vi "SL TAGS Write Server Tag.vi"(8 "error in (no error)":errorcluster, 10 "Value":variant, 11 "Tag Ref In":T1) -> (0 "error out":errorcluster, 3 "Tag Ref Out":T1)   [LabVIEW 2017, in "EEISysLink.lvclass"]
doc: "Will input a class tag and write its value to the SystemLink server. \n\nNote: this does not update the local class tag value. You must read from the server to get the value. \n\nJames Tillett P.E.\nEndeavor Engineering Inc.\nwww.endeavoreng.com"
uses:
  EEISysLink.lvclass
  Controls/SL Tag.ctl
  <vilib>/Skyline/Tag/Wrapper/Wrapper_class/NI Skyline Tag.lvclass
  Controls/SL Tag Properties.ctl
  Controls/SL Tag Data Type.ctl
  Controls/SL Tag Interpolation Method.ctl
  Controls/SL Tag Unit of Measure.ctl
  Controls/SL Tag Type.ctl
  <vilib>/Skyline/Tag/Shared/typedefs/Tag Cluster.ctl
  <vilib>/Skyline/Tag/Shared/typedefs/DataType.ctl
  <vilib>/Skyline/Tag/Wrapper/Wrapper_class/Write Tag (DBL).vi
  <vilib>/Skyline/Tag/Wrapper/Wrapper_class/Write Tag (I32).vi
  <vilib>/Skyline/Tag/Wrapper/Wrapper_class/Write Tag (String).vi
  <vilib>/Skyline/Tag/Shared/NI Skyline Tag.lvlib
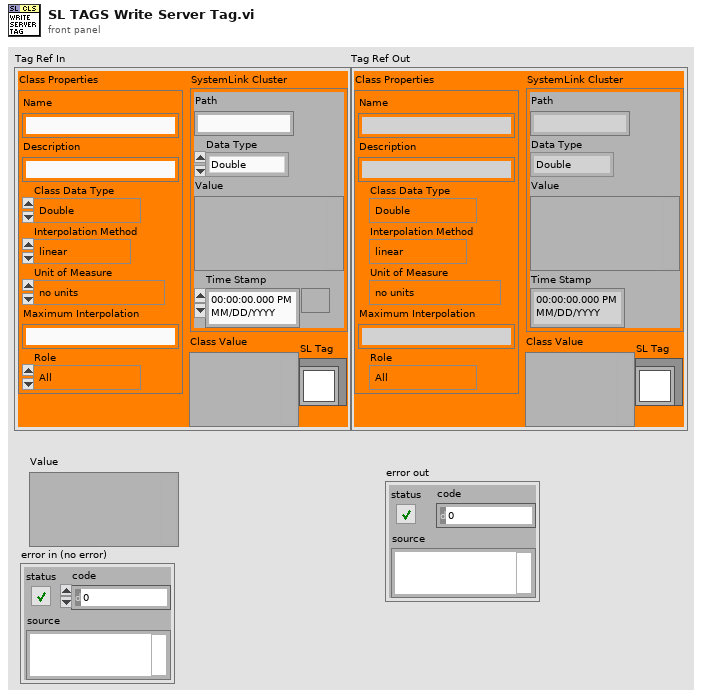
[diagram p1: front panel]
types:
  T1 = typedef "EEISysLink.lvclass/SL Tag.ctl" = cluster{"Class Properties":T2, "SL Tag":refnum<class "NI Skyline Tag.lvclass">, "SystemLink Cluster":T7, "Class Value":variant}
  T2 = typedef "EEISysLink.lvclass/SL Tag Properties.ctl" = cluster{"Class Data Type":T3, "Name":string, "Description":string, "Interpolation Method":T4, "Unit of Measure":T5, "Maximum Interpolation":string, "Role":T6}
  T3 = typedef "EEISysLink.lvclass/SL Tag Data Type.ctl" = enum16{"Double", "Integer", "String", "Boolean", "Waveform"}
  T4 = typedef "EEISysLink.lvclass/SL Tag Interpolation Method.ctl" = enum16{"linear", "pilinear", "step"}
  T5 = typedef "EEISysLink.lvclass/SL Tag Unit of Measure.ctl" = enum16{"no units", "Second", "Hour", "Minute", "Day", "Year", "Month", "Week", "Foot", "Yard", "Meter", "Centimeter", "Inch", "Mile", "Nautical Mile", "Miles per Hour", "Meters per second", "Square meter", "Cubic meter", "Cubic centimeter", "Cubic inch", "Liter", "Gallon", "Gallons dry US", "Gallon UK", "Percent", "Revolutions per minute", "Revolution", "Degree angle", "Astronomical Unit", "Atom", "Atomic mass", "Bar", "Byte", "C (speed of light)", "Curie", "Decibel", "Electron Volt", "Ounce", "Knot", "G", "Grade", "Are", "Hectare", "Faraday", "Franklin", "Gilbert", "Erg", "Lambert", "Maxwell", "Gauss", "Electron mass", "Kilogram force", "Pound force", "Rad", "Centiradian", "Sphere", "Mach", "Fluid Ounces", "Fluid Ounces UK", "Fahrenheit", "Celsius", "Kelvin", "Rankine", "Gram", "Kilogram", "Pound", "Short/US Ton", "Long/UK ton", "Metric ton", "Mole", "Pounds per square inch", "Inches water column", "Torr", "Millitorr", "Millimeter mercury", "Inches mercury", "Bar (2)", "Atmosphere", "Pascal", "Watt", "kiloWatt", "Horsepower", "Kilowatt Hour", "British thermal units", "Millions of BTU", "Ampere", "Candela", "Radian", "Steradian", "Bit", "Hertz", "Newton", "Joule", "Coulomb", "Volt", "Farad", "Ohm", "Siemens", "Weber", "Tesla", "Henry", "Lumen", "Lux", "Becqueral", "Gray", "Sievert", "Katal", "Angstrom", "Light Year", "Parsec", "Point", "Pixel", "Dyne", "Kilogram force (2)", "Pound force (2)", "Rem", "Rutherford", "Roentgen"}
  T6 = typedef "EEISysLink.lvclass/SL Tag Type.ctl" = enum16{"All", "Supervisor", "Worker"}
  T7 = typedef "NI Skyline Tag.lvlib/Tag Cluster.ctl" = cluster{"Path":string, "Data Type":T8, "Value":variant, "Time Stamp":timestamp}
  T8 = typedef "NI Skyline Tag.lvlib/DataType.ctl" = enum32{"Double", "Integer", "String"}
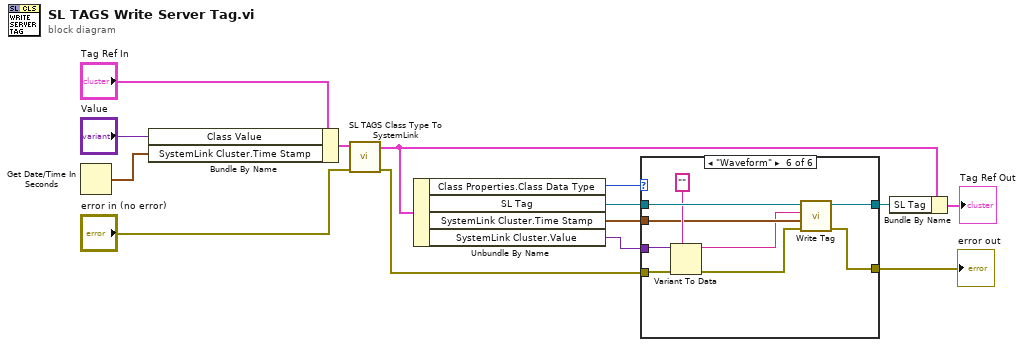
[diagram p0: block diagram]
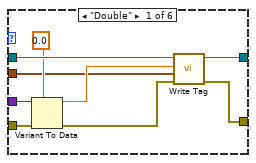
[diagram p2: hidden frame]
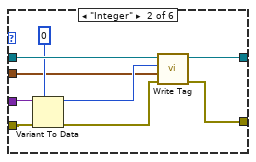
[diagram p3: hidden frame]
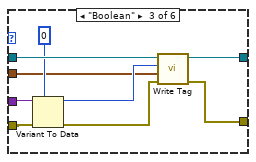
[diagram p4: hidden frame]
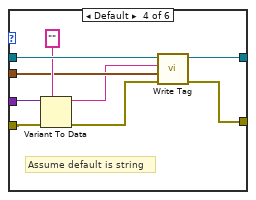
[diagram p5: hidden frame]
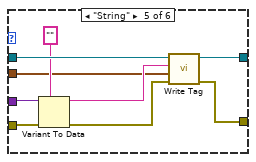
[diagram p6: hidden frame]
diagram:
  n1 = Get Date/Time In Seconds() -> (seconds since 1Jan1904=w7:timestamp)
  n2 = Bundle By Name(cluster="Tag Ref In", "Class Value"="Value", "SystemLink Cluster.Time Stamp"=w7) -> (w6:T1)
  n3 = call "SL TAGS Class Type To SystemLink.vi"("error in (no error)"="error in (no error)", "Class Tag In"=w6) -> ("error out"=w3:errorcluster, "Class Tag Out"=w2:T1)  [unwired: 7 in, 1 out]
  n4 = Unbundle By Name(w2) -> ("Class Properties.Class Data Type"=w14:T3, "SL Tag"=w11:refnum<class "NI Skyline Tag.lvclass">, "SystemLink Cluster.Time Stamp"=w1:timestamp, "SystemLink Cluster.Value"=w4:variant)
  n5 = case shown="\"Waveform\"" w14 {
    tunnel: [w23 w32 w41 w50 w59 w68] -> w12
    tunnel: [w22 w31 w40 w49 w58 w67] -> w10
    tunnel: w3 -> [w19 w27 w36 w46 w54 w63]
    tunnel: w11 -> [w21 w30 w39 w48 w57 w66]
    tunnel: w4 -> [w18 w28 w37 w47 w55 w64]
    tunnel: w1 -> [w15 w24 w33 w43 w51 w61]
    frame "Double" {
      n6 = Variant To Data(error in=w19, type=0.0, Variant=w18) -> (data=w16:dbl, error out=w17:errorcluster)
      n7 = call-poly <vilib>:"Write Tag.vi"("error in (no error)"=w17, "time stamp"=w15, "value"=w16, "tag in"=w21) -> ("error out"=w22:errorcluster, "tag out"=w23:refnum<class "NI Skyline Tag.lvclass">)  [unwired: 6 in]
    }
    frame "Integer" {
      n8 = Variant To Data(error in=w27, type=0, Variant=w28) -> (data=w25:i32, error out=w26:errorcluster)
      n9 = call-poly <vilib>:"Write Tag.vi"("error in (no error)"=w26, "time stamp"=w24, "value"=w25, "tag in"=w30) -> ("error out"=w31:errorcluster, "tag out"=w32:refnum<class "NI Skyline Tag.lvclass">)  [unwired: 6 in]
    }
    frame "Boolean" {
      n10 = Variant To Data(error in=w36, type=0, Variant=w37) -> (data=w34:i32, error out=w35:errorcluster)
      n11 = call-poly <vilib>:"Write Tag.vi"("error in (no error)"=w35, "time stamp"=w33, "value"=w34, "tag in"=w39) -> ("error out"=w40:errorcluster, "tag out"=w41:refnum<class "NI Skyline Tag.lvclass">)  [unwired: 6 in]
    }
    frame Default {
      # "Assume default is string"
      n12 = Variant To Data(error in=w46, type="", Variant=w47) -> (data=w42:string, error out=w44:errorcluster)
      n13 = call-poly <vilib>:"Write Tag.vi"("error in (no error)"=w44, "time stamp"=w43, "value"=w42, "tag in"=w48) -> ("error out"=w49:errorcluster, "tag out"=w50:refnum<class "NI Skyline Tag.lvclass">)  [unwired: 6 in]
    }
    frame "String" {
      n14 = Variant To Data(error in=w54, type="", Variant=w55) -> (data=w52:string, error out=w53:errorcluster)
      n15 = call-poly <vilib>:"Write Tag.vi"("error in (no error)"=w53, "time stamp"=w51, "value"=w52, "tag in"=w57) -> ("error out"=w58:errorcluster, "tag out"=w59:refnum<class "NI Skyline Tag.lvclass">)  [unwired: 6 in]
    }
    frame "Waveform" {
      n16 = Variant To Data(error in=w63, type="", Variant=w64) -> (data=w60:string, error out=w62:errorcluster)
      n17 = call-poly <vilib>:"Write Tag.vi"("error in (no error)"=w62, "time stamp"=w61, "value"=w60, "tag in"=w66) -> ("error out"=w67:errorcluster, "tag out"=w68:refnum<class "NI Skyline Tag.lvclass">)  [unwired: 6 in]
    }
  }
  "error out" <- w10
  n18 = Bundle By Name(cluster=w2, "SL Tag"=w12) -> (→"Tag Ref Out":T1)
